vi "exchange rate.vi"() -> ()   [LabVIEW 2014]
uses:
  <vilib>/Utility/file.llb/Write To Spreadsheet File (string).vi
  <vilib>/regexp/Match Regular Expression.xnode
  <vilib>/httpClient/LabVIEWHTTPClient.lvlib
panel:
  out "웨이브폼 그래프":i32[](graph)
  out "현재 환율 2":string
  in  "확인 버튼":bool
  in  "world":string(combo)="USD"
  in  "day":string(combo)="13"
  in  "month":string(combo)="08"
  in  "year":string(combo)="2018"
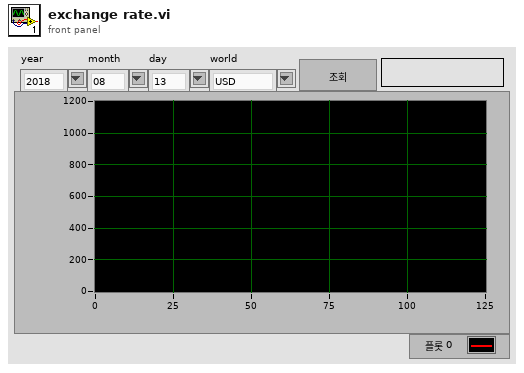
[diagram p1: front panel]
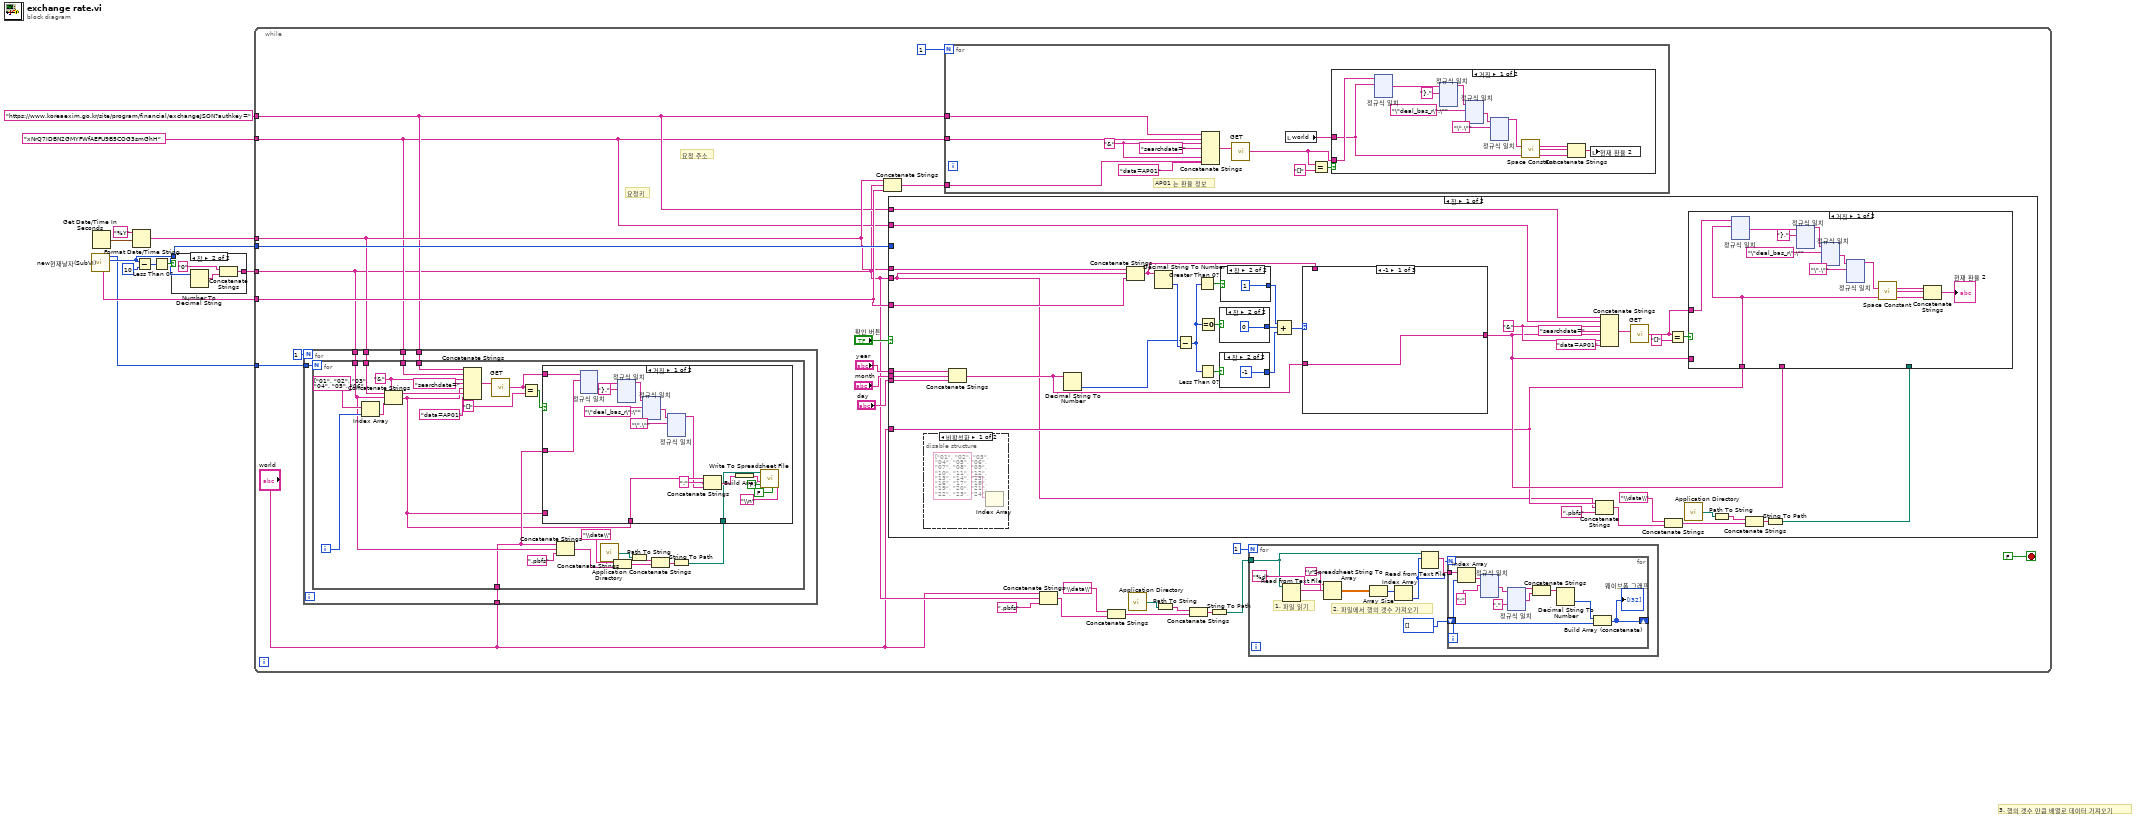
[diagram p0: block diagram]
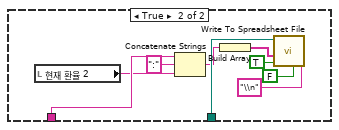
[diagram p2: hidden frame]
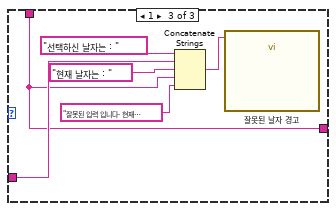
[diagram p6: hidden frame]
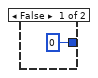
[diagram p7: hidden frame]
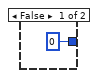
[diagram p8: hidden frame]
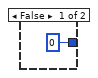
[diagram p9: hidden frame]
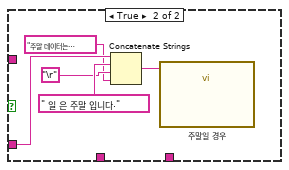
[diagram p10: hidden frame]
diagram:
  # "3. 행의 갯수 만큼 배열로 데이터 가져오기"
  n1 = call "new현재날자(SubVI).vi"() -> ("월"=w6:i32, "일"=w1:i32, "일 문자열"=w5:string)  [unwired: 5 in, 4 out]
  n2 = Get Date/Time In Seconds() -> (seconds since 1Jan1904=w9:timestamp)
  n3 = Format Date/Time String(time format string (%c)="%Y" ("시간 포맷 문자열 (%c)"), seconds (now)=w9) -> (date/time string=w7:string)  [unwired: 1 in]
  n4 = Subtract(x=w6, y=10) -> (x-y=w11:i32)
  n5 = Less Than 0?(x=w11) -> (x < 0?=w10:bool)
  n6 = case shown="참" w10 {
    tunnel: w6 -> [_ w16]
    tunnel: [_ w13] -> w4
    frame False {
    }
    frame True {
      n7 = Number To Decimal String(number=w16) -> (decimal integer string=w15:string)  [unwired: 1 in]
      n8 = Concatenate Strings("0", w15) -> (w13:string)
    }
  }
  n9 = while {
    tunnel: w7 -> [w22]
    tunnel: w6 -> [w25]
    tunnel: w5 -> [w24]
    tunnel: w4 -> [w19]
    tunnel: "https://www.koreaexim.go.kr/site/program/financial/exchangeJSON?authkey=" -> [w21]
    tunnel: "xNrQ7IDBN2GMYFWfAEFU9B5COG3smGhH" -> [w20]
    tunnel: w1 -> [w23]
    stop <- FALSE stop-if-true
    # "요청 주소"
    # "요청키"
    n10 = for {
      N: 1 -> [_]
      tunnel: w23 -> [w47]
      tunnel: w22 -> [w46]
      tunnel: w21 -> [w45]
      tunnel: w20 -> [w44]
      tunnel: w19 -> [w43]
      tunnel: "world" -> [w42]
      n11 = for {
        N: w47 -> [_]
        tunnel: w46 -> [w66]
        tunnel: w45 -> [w68]
        tunnel: w44 -> [w67]
        tunnel: w43 -> [w50]
        tunnel: w42 -> [w49]
        i -> [w63]
        w70 = "&" ("문자열")
        n12 = Index Array(array=string[] ["01", "02", "03", "04", "05", "06", "07", "08", "09", "10", "11", "12", "13", "14", "15", "16", "17", "18", "19", "20", "21", "22", "23", "24", "25", "26", "27", "28", "29", "30", "31"], index=w63) -> (element=w64:string)
        n13 = Concatenate Strings(w66, w50, w64) -> (w48:string)
        n14 = Concatenate Strings(w68, w67, w70, "searchdate=" ("문자열"), w48, w70, "data=AP01" ("문자열")) -> (w61:string)
        n15 = call <vilib>:"GET.vi"("url"=w61) -> ("body"=w59:string)  [unwired: 11 in, 3 out]
        n16 = Equal?(x=w59, y="[]") -> (x = y?=w60:bool)
        n17 = Concatenate Strings(w49, w50, ".pbfs" ("문자열")) -> (w53:string)
        n18 = call <vilib>:"Application Directory.vi"() -> ("Application Directory"=w56:path)
        n19 = Concatenate Strings("\\data\\" ("문자열"), w53) -> (w52:string)
        n20 = Path To String(path=w56) -> (string=w58:string)
        n21 = Concatenate Strings(w58, w52) -> (w57:string)
        n22 = String To Path(string=w57) -> (path=w51:path)
        n23 = case shown="거짓" w60 {
          tunnel: w48 -> [_ _]
          tunnel: w59 -> [w82 _]
          tunnel: w48 -> [w75 w547]
          tunnel: w51 -> [w73 w549]
          tunnel: w49 -> [w72 _]
          frame False {
            n24 = xnode ("정규식 일치")("입력 문자열"=w82, "정규식"=w72) -> ("일치 구문 뒤"=w83:string)  [unwired: 4 in, 4 out]
            n25 = xnode ("정규식 일치")("입력 문자열"=w83, "정규식"="},") -> ("일치 구문 앞"=w85:string)  [unwired: 4 in, 4 out]
            n26 = xnode ("정규식 일치")("입력 문자열"=w85, "정규식"="\"deal_bas_r\":\"") -> ("일치 구문 뒤"=w87:string)  [unwired: 4 in, 4 out]
            n27 = xnode ("정규식 일치")("입력 문자열"=w87, "정규식"="\",\"") -> ("일치 구문 앞"=w74:string)  [unwired: 4 in, 4 out]
            n28 = Concatenate Strings(w75, ":", w74) -> (w77:string)
            n29 = Build Array(w77) -> (w78:string[])
            n30 = call-poly <vilib>:"Write To Spreadsheet File.vi"("delimiter (\\t)"="\\n" ("delimiter (\\t)"), "transpose? (no:F)"=FALSE, "append to file? (new file:F)"=TRUE, "1D data"=w78, "file path (dialog if empty)"=w73) -> ()  [unwired: 3 in, 1 out]
          }
          frame True {
            n31 = local read "현재 환율 2"() -> (w546:string)
            n32 = Concatenate Strings(w547, ":", w546) -> (w545:string)
            n33 = Build Array(w545) -> (w550:string[])
            n34 = call-poly <vilib>:"Write To Spreadsheet File.vi"("delimiter (\\t)"="\\n" ("delimiter (\\t)"), "transpose? (no:F)"=FALSE, "append to file? (new file:F)"=TRUE, "1D data"=w550, "file path (dialog if empty)"=w549) -> ()  [unwired: 3 in, 1 out]
          }
        }
      }
    }
    n35 = Concatenate Strings(w22, w19, w24) -> (w30:string)
    n36 = case shown="참" "확인 버튼" {
      tunnel: "world" -> [w1290 _]
      tunnel: w24 -> [w1289 _]
      tunnel: w22 -> [w1288 _]
      tunnel: w19 -> [w1281 _]
      tunnel: "month" -> [w1285 _]
      tunnel: "day" -> [w1286 _]
      tunnel: "year" -> [w1284 _]
      tunnel: w25 -> [_ _]
      tunnel: w21 -> [w1283 _]
      tunnel: w20 -> [w1282 _]
      frame True {
        w1316 = "&" ("문자열")
        n37 = disable-structure shown="비활성화" {
          frame Disabled {
            n38 = Index Array(array=string[] ["01", "02", "03", "04", "05", "06", "07", "08", "09", "10", "11", "12", "13", "14", "15", "16", "17", "18", "19", "20", "21", "22", "23", "24", "25", "26", "27", "28", "29", "30", "31"]) -> ()  [unwired: 1 in, 1 out]
          }
          frame Enabled {
          }
        }
        n39 = Concatenate Strings(w1284, w1285, w1286) -> (w1287:string)
        n40 = Decimal String To Number(string=w1287) -> (number=w1309:i32)  [unwired: 2 in, 1 out]
        n41 = Concatenate Strings(w1288, w1281, w1289) -> (w1300:string)
        n42 = Decimal String To Number(string=w1300) -> (number=w1310:i32)  [unwired: 2 in, 1 out]
        n43 = Subtract(x=w1309, y=w1310) -> (x-y=w1305:i32)
        n44 = Greater Than 0?(x=w1305) -> (x > 0?=w1306:bool)
        n45 = Less Than 0?(x=w1305) -> (x < 0?=w1308:bool)
        n46 = Equal To 0?(x=w1305) -> (x = 0?=w1307:bool)
        n47 = case shown="참" w1308 {
          tunnel: [0 -1] -> w1302
          frame False {
          }
          frame True {
          }
        }
        n48 = case shown="참" w1307 {
          tunnel: [0 0] -> w1303
          frame False {
          }
          frame True {
          }
        }
        n49 = case shown="참" w1306 {
          tunnel: [0 1] -> w1304
          frame False {
          }
          frame True {
          }
        }
        n50 = Compound Arithmetic op=ADD(w1304, w1303, w1302) -> (w1301:i32)
        n51 = case shown="-1" w1301 {
          tunnel: w1287 -> [w1319 _ w1325]
          tunnel: w1300 -> [_ w1320 w1323]
          tunnel: [w1319 w1320 w1323] -> w1292
          frame -1 {
          }
          frame 0, Default {
          }
          frame 1 {
            n52 = Concatenate Strings("선택하신 날자는 : " ("문자열"), w1325, "현재 날자는 : ", w1323, "잘못된 입력 입니다. 현재 날자로 검색을 진행 합니다." ("문자열")) -> (w1321:string)
            n53 = call "잘못된 날자 경고"("Message"=w1321) -> ()  [unwired: 9 in, 2 out]
          }
        }
        n54 = Concatenate Strings(w1290, w1281, ".pbfs" ("문자열")) -> (w1294:string)
        n55 = Concatenate Strings(w1283, w1282, w1316, "searchdate=" ("문자열"), w1292, w1316, "data=AP01" ("문자열")) -> (w1314:string)
        n56 = call <vilib>:"GET.vi"("url"=w1314) -> ("body"=w1311:string)  [unwired: 11 in, 3 out]
        n57 = Concatenate Strings("\\data\\" ("문자열"), w1294) -> (w1293:string)
        n58 = Equal?(x=w1311, y="[]") -> (x = y?=w1312:bool)
        n59 = call <vilib>:"Application Directory.vi"() -> ("Application Directory"=w1297:path)
        n60 = Path To String(path=w1297) -> (string=w1299:string)
        n61 = Concatenate Strings(w1299, w1293) -> (w1298:string)
        n62 = String To Path(string=w1298) -> (path=w1291:path)
        n63 = case shown="거짓" w1312 {
          tunnel: w1292 -> [_ w1804]
          tunnel: w1311 -> [w1335 _]
          tunnel: w1290 -> [w1334 _]
          tunnel: w1292 -> [_ _]
          tunnel: w1291 -> [_ _]
          frame False {
            n64 = xnode ("정규식 일치")("입력 문자열"=w1335, "정규식"=w1334) -> ("일치 구문 뒤"=w1336:string)  [unwired: 4 in, 4 out]
            n65 = xnode ("정규식 일치")("입력 문자열"=w1336, "정규식"="},") -> ("일치 구문 앞"=w1338:string)  [unwired: 4 in, 4 out]
            n66 = xnode ("정규식 일치")("입력 문자열"=w1338, "정규식"="\"deal_bas_r\":\"") -> ("일치 구문 뒤"=w1340:string)  [unwired: 4 in, 4 out]
            n67 = xnode ("정규식 일치")("입력 문자열"=w1340, "정규식"="\",\"") -> ("일치 구문 앞"=w1333:string)  [unwired: 4 in, 4 out]
            n68 = call <vilib>:"Space Constant.vi"() -> ("String"=w1342:string)
            n69 = Concatenate Strings(w1333, w1342, w1334) -> (→"현재 환율 2":string)
          }
          frame True {
            n70 = Concatenate Strings(w1804, " 일 은 주말 입니다.", "\r", "주말 데이터는 제공되지 않습니다.") -> (w1800:string)
            n71 = call "주말일 경우"("Message"=w1800) -> ()  [unwired: 9 in, 2 out]
          }
        }
      }
      frame False {
      }
    }
    n72 = for {
      N: 1 -> [_]
      tunnel: w30 -> [w560]
      tunnel: w21 -> [w555]
      tunnel: w20 -> [w554]
      w562 = "&" ("문자열")
      # "AP01 는 환율 정보"
      n73 = Concatenate Strings(w555, w554, w562, "searchdate=" ("문자열"), w560, w562, "data=AP01" ("문자열")) -> (w564:string)
      n74 = call <vilib>:"GET.vi"("url"=w564) -> ("body"=w556:string)  [unwired: 11 in, 3 out]
      n75 = local read "world"() -> (w559:string)
      n76 = Equal?(x=w556, y="[]") -> (x = y?=w557:bool)
      n77 = case shown="거짓" w557 {
        tunnel: w556 -> [w568 _]
        tunnel: w559 -> [w566 _]
        frame False {
          n78 = xnode ("정규식 일치")("입력 문자열"=w568, "정규식"=w566) -> ("일치 구문 뒤"=w569:string)  [unwired: 4 in, 4 out]
          n79 = xnode ("정규식 일치")("입력 문자열"=w569, "정규식"="},") -> ("일치 구문 앞"=w571:string)  [unwired: 4 in, 4 out]
          n80 = xnode ("정규식 일치")("입력 문자열"=w571, "정규식"="\"deal_bas_r\":\"") -> ("일치 구문 뒤"=w573:string)  [unwired: 4 in, 4 out]
          n81 = xnode ("정규식 일치")("입력 문자열"=w573, "정규식"="\",\"") -> ("일치 구문 앞"=w567:string)  [unwired: 4 in, 4 out]
          n82 = call <vilib>:"Space Constant.vi"() -> ("String"=w575:string)
          n83 = Concatenate Strings(w567, w575, w566) -> (w565:string)
          n84 = local write "현재 환율 2"(w565) -> ()
        }
        frame True {
        }
      }
    }
    n85 = Concatenate Strings("world", w19, ".pbfs" ("문자열")) -> (w37:string)
    n86 = Concatenate Strings("\\data\\" ("문자열"), w37) -> (w38:string)
    n87 = call <vilib>:"Application Directory.vi"() -> ("Application Directory"=w34:path)
    n88 = Path To String(path=w34) -> (string=w32:string)
    n89 = Concatenate Strings(w32, w38) -> (w33:string)
    n90 = String To Path(string=w33) -> (path=w31:path)
    n91 = for {
      N: 1 -> [_]
      tunnel: w31 -> [w1033]
      # "2. 파일에서 행의 갯수 가져오기"
      # "1. 파일 읽기"
      n92 = Read from Text File(file (use dialog)=w1033) -> (text=w1040:string)  [unwired: 1 in, 5 out]
      n93 = Spreadsheet String To Array(delimiter (Tab)="\r", format string="%d", spreadsheet string=w1040) -> (array=w1038:dbl[][])  [unwired: 1 out]
      n94 = Array Size(array=w1038) -> (size(s)=w1039:i32[])
      n95 = Index Array(array=w1039) -> (element=w1034:i32)  [unwired: 1 in]
      n96 = Read from Text File(file (use dialog)=w1033, count=w1034) -> (text=w1035:string[])  [unwired: 1 in, 4 out]
      n97 = for {
        N: w1034 -> [_]
        tunnel: w1035 -> [w1044]
        shift-right: [w1041] -> _
        shift-left: i32[] [] -> [w1043]
        i -> [w1045]
        n98 = Index Array(array=w1044, index=w1045) -> (element=w1052:string)
        n99 = xnode "정규식 일치"("입력 문자열"=w1052, "정규식"=":") -> ("일치 구문 뒤"=w1050:string)  [unwired: 4 in, 4 out]
        n100 = xnode "정규식 일치"("입력 문자열"=w1050, "정규식"=",") -> ("일치 구문 앞"=w1048:string, "일치 구문 뒤"=w1047:string)  [unwired: 4 in, 3 out]
        n101 = Concatenate Strings(w1048, w1047) -> (w1046:string)
        n102 = Decimal String To Number(string=w1046) -> (number=w1042:i32)  [unwired: 2 in, 1 out]
        n103 = Build Array (concatenate)(w1042, w1043) -> (w1041:i32[])
        "웨이브폼 그래프" <- w1041
      }
    }
  }
